vi "Get CEID Data.vi"(8 "error in":errorcluster, 11 "CEID":u32) -> (0 "error out":errorcluster, 2 "Find?":bool, 3 "CEID Data":T1)   [LabVIEW 2020, in "SECS Communication.lvlib" / "SECS Data Class.lvclass"]
uses:
  SECS Data Class.lvclass
  CEID Data.ctl
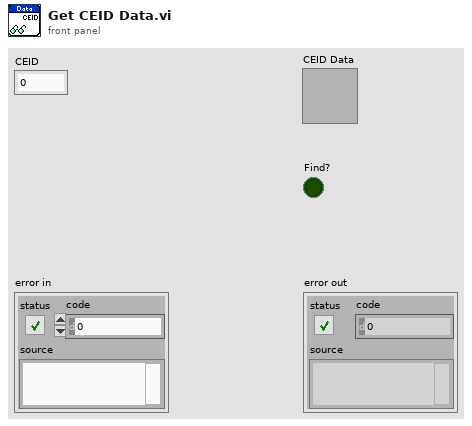
[diagram p1: front panel]
types:
  T1 = typedef "SECS Communication.lvlib/SECS Data Class.lvclass/CEID Data.ctl" = cluster{"Enable":bool, "CEID":u32, "Name":string, "Description":string, "RPTID":u32[], "Dynamic":bool}
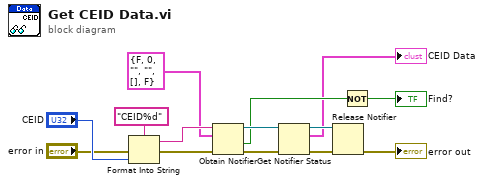
[diagram p0: block diagram]
diagram:
  n1 = Format Into String(format string="CEID%d", error in="error in", "CEID") -> (resulting string=w9:string, error out=w10:errorcluster)  [unwired: 1 in]
  n2 = Obtain Notifier(name (unnamed)=w9, notification data type=T1 {"Enable"=FALSE, "CEID"=0, "Name"="", "Description"="", "RPTID"=[], "Dynamic"=FALSE} ("CEID Data"), error in (no error)=w10) -> (notifier out=w14:refnum<notifier>, created new?=w5:bool, error out=w3:errorcluster)  [unwired: 1 in]
  n3 = Get Notifier Status(notifier=w14, error in (no error)=w3) -> (notifier out=w13:refnum<notifier>, current notification=→"CEID Data":T1, error out=w12:errorcluster)  [unwired: 2 out]
  n4 = Release Notifier(notifier=w13, error in (no error)=w12) -> (error out=→"error out":errorcluster)  [unwired: 1 in, 2 out]
  n5 = Not(x=w5) -> (.not. x?=→"Find?":bool)
